vi "Launch Asynchronous Logging Loop.vi"(6 "Log Status FIFO":refnum<k33>, 8 "error in (no error)":errorcluster, 9 "Log Data FIFO Size":i32, 10 "Log Data FIFO":refnum<k33>, 11 "File Logging Specs":T1[](array[typedef]) {"File Node Ref" format="%.0x"}) -> (0 "error out":errorcluster)   [LabVIEW 2027, in "Embedded Data Logger Engine.lvlib"]
uses:
  Embedded Data Logger Engine.lvlib
  File Logging Specification.ctl
  Group Logging Specification.ctl
  Group Buffer Data.ctl
  Property Specification.ctl
  <vilib>/NI VeriStand/Custom Device API/Custom Device Item Ref.ctl
  Shared/Segment Files By.ctl
  Logging State.ctl
  <vilib>/NI VeriStand/Custom Device API/Custom Device API.lvlib
  Shared/Embedded Data Logger Shared.lvlib
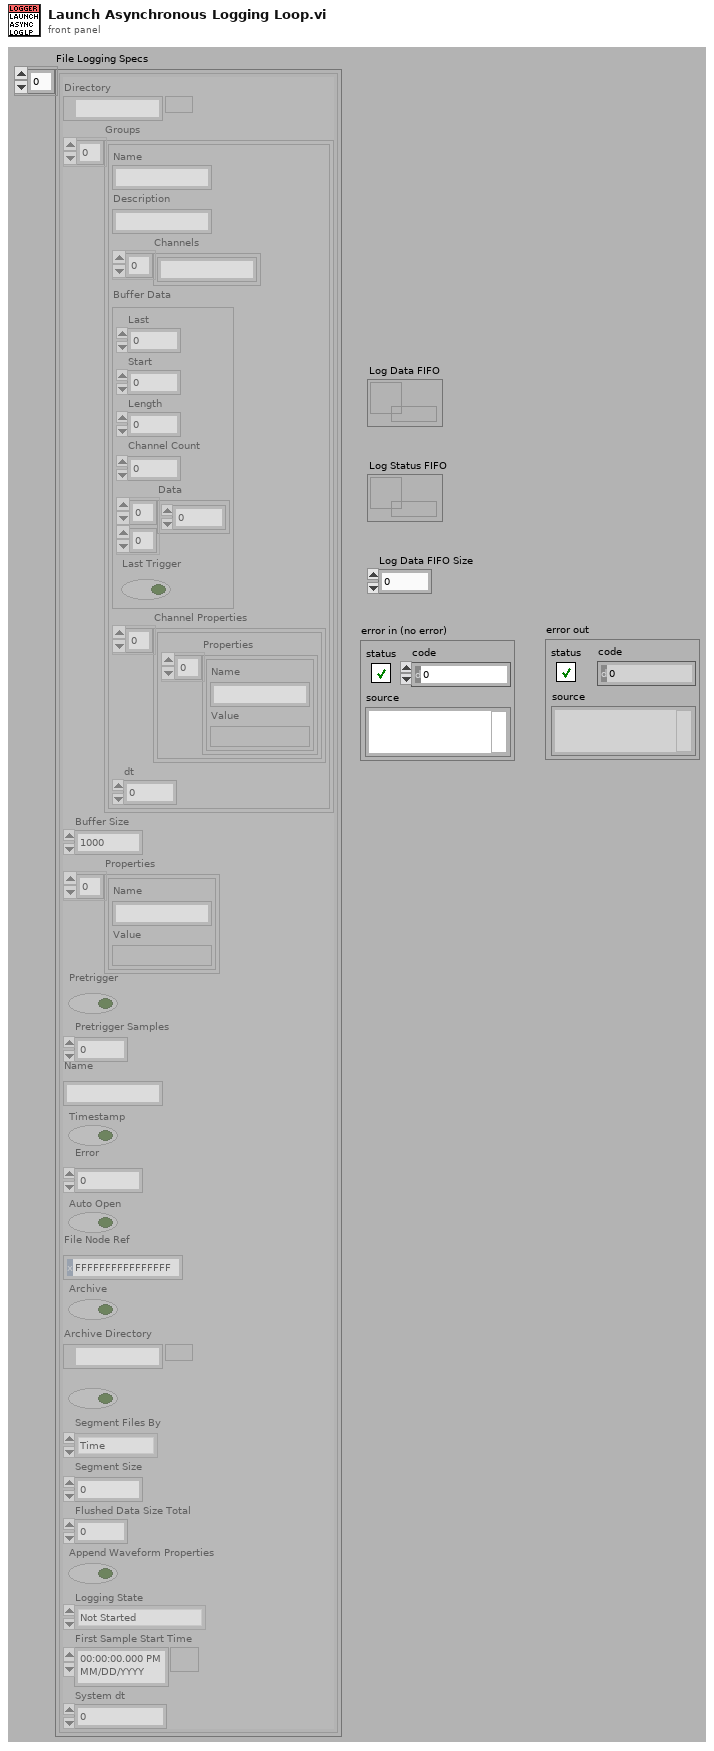
[diagram p1: front panel]
types:
  T1 = typedef "Embedded Data Logger Engine.lvlib/File Logging Specification.ctl" = cluster{"Directory":path, "Groups":T2[], "Buffer Size":i32, "Properties":T4[], "Pretrigger":bool, "Pretrigger Samples":i32, "Name":string, "Timestamp":bool, "Error":i32, "Auto Open":bool, "File Node Ref":T5, "Archive":bool, "Archive Directory":path, "Segment Files":bool, "Segment Files By":T6, "Segment Size":u32, "Flushed Data Size Total":u32, "Append Waveform Properties":bool, "Logging State":T7, "First Sample Start Time":timestamp, "System dt":dbl}
  T2 = typedef "Embedded Data Logger Engine.lvlib/Group Logging Specification.ctl" = cluster{"Name":string, "Description":string, "Channels":string[], "Buffer Data":T3, "Channel Properties":cluster{"Properties":T4[]}[], "dt":dbl}
  T3 = typedef "Embedded Data Logger Engine.lvlib/Group Buffer Data.ctl" = cluster{"Last":i32, "Start":i32, "Length":i32, "Channel Count":i32, "Data":dbl[][], "Last Trigger":bool}
  T4 = typedef "Embedded Data Logger Engine.lvlib/Property Specification.ctl" = cluster{"Name":string, "Value":variant}
  T5 = typedef "Custom Device API.lvlib/Custom Device Item Ref.ctl" = u64
  T6 = typedef "Embedded Data Logger Shared.lvlib/Segment Files By.ctl" = enum16{"Time", "Size"}
  T7 = typedef "Embedded Data Logger Engine.lvlib/Logging State.ctl" = enum16{"Not Started", "Continous Logging", "Paused", "Discontinous Logging"}
  T8 = cluster{"Log Data FIFO Size":i32, "Log Status FIFO":refnum<k33>, "Log Data FIFO":refnum<k33>, "File Logging Specs":T1[]}
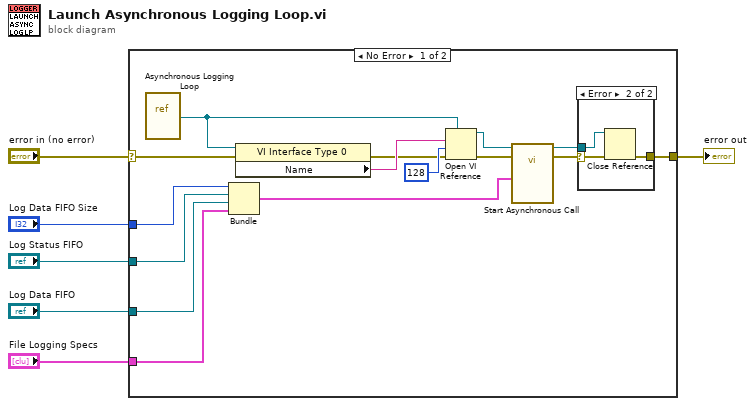
[diagram p0: block diagram]
diagram:
  n1 = case shown="No Error" "error in (no error)" {
    selector: "error in (no error)" -> [w9 w26]
    tunnel: [w20 w26] -> w6
    tunnel: "Log Data FIFO Size" -> [w19 _]
    tunnel: "Log Status FIFO" -> [w18 _]
    tunnel: "Log Data FIFO" -> [w17 _]
    tunnel: "File Logging Specs" -> [w16 _]
    frame No Error {
      n2 = vi-ref "Asynchronous Logging Loop.vi"() -> (w7:refnum<vi>)
      n3 = Bundle("Log Data FIFO Size"=w19, "Log Status FIFO"=w18, "Log Data FIFO"=w17, "File Logging Specs"=w16) -> (w13:T8)  [unwired: 1 out]
      n4 = property class="VI Interface Type 0"(reference=w7, error in=w9) -> (error out=w8:errorcluster, "Name"=w21:string)  [unwired: 1 out]
      n5 = Open VI Reference(type specifier VI Refnum (for type only)=w7, vi path=w21, options=128, error in (no error)=w8) -> (vi reference=w14:refnum<vi>, error out=w15:errorcluster)  [unwired: 2 out]
      n6 = call-by-ref "Start Asynchronous Call"(reference=w14, error in=w15, "Input Data"=w13) -> (reference out=w11:refnum<vi>, error out=w12:errorcluster)  [unwired: 11 in]
      n7 = case shown="Error" w12 {
        selector: w12 -> [w22 w25]
        tunnel: w11 -> [_ w24]
        tunnel: [w22 w23] -> w20
        frame No Error {
        }
        frame Error {
          n8 = Close Reference(reference=w24, error in (no error)=w25) -> (error out=w23:errorcluster)
        }
      }
    }
    frame Error {
    }
  }
  "error out" <- w6
